vi "Decimal Rounding.vi"(8 "Round Method (Nearest)":T1(ring)=enum."Round Nearest", 10 "Digits past \".\" (1)":i32=1, 11 "Input":dbl format="%#_13g") -> (3 "Output":dbl format="%#_13g")   [LabVIEW 2022 SP3]
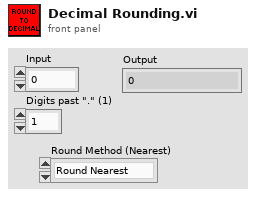
[diagram p1: front panel]
types:
  T1 = enum16{"Round to +INF", "Round Nearest", "Round to -INF"}
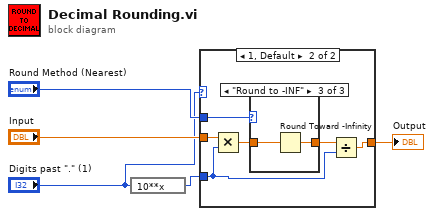
[diagram p0: block diagram]
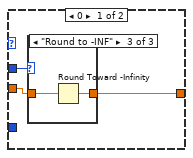
[diagram p2: hidden frame]
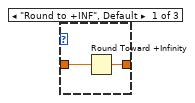
[diagram p3: hidden frame]
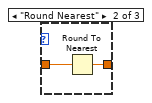
[diagram p4: hidden frame]
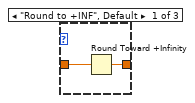
[diagram p5: hidden frame]
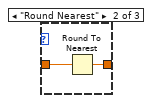
[diagram p6: hidden frame]
diagram:
  n1 = expression code="10**x"("Digits past \".\" (1)") -> (w1:i32)
  n2 = case shown="1, Default" "Digits past \".\" (1)" {
    tunnel: "Input" -> [w7 w20]
    tunnel: "Round Method (Nearest)" -> [w6 w19]
    tunnel: [w8 w17] -> w3
    tunnel: w1 -> [_ w15]
    frame 0 {
      n3 = case shown="\"Round to -INF\"" w6 {
        tunnel: [w9 w11 w13] -> w8
        tunnel: w7 -> [w10 w12 w14]
        frame "Round to +INF", Default {
          n4 = Round Toward +Infinity(x=w10) -> (ceil(x): smallest int >= x=w9:dbl)
        }
        frame "Round Nearest" {
          n5 = Round To Nearest(number=w12) -> (nearest integer value=w11:dbl)
        }
        frame "Round to -INF" {
          n6 = Round Toward -Infinity(1:w14) -> (0:w13:dbl)
        }
      }
    }
    frame 1, Default {
      n7 = Multiply(x=w20, y=w15) -> (x*y=w18:dbl)
      n8 = case shown="\"Round to -INF\"" w19 {
        tunnel: [w21 w23 w25] -> w16
        tunnel: w18 -> [w22 w24 w26]
        frame "Round to +INF", Default {
          n9 = Round Toward +Infinity(x=w22) -> (ceil(x): smallest int >= x=w21:dbl)
        }
        frame "Round Nearest" {
          n10 = Round To Nearest(number=w24) -> (nearest integer value=w23:dbl)
        }
        frame "Round to -INF" {
          n11 = Round Toward -Infinity(1:w26) -> (0:w25:dbl)
        }
      }
      n12 = Divide(x=w16, y=w15) -> (x/y=w17:dbl)
    }
  }
  "Output" <- w3
